vi "Cleanup.vi"(8 "error in (no error)":errorcluster, 11 "PlatformArrayPanel in":refnum<class "PlatformArrayPanel.lvclass">) -> (0 "error out":errorcluster)   [LabVIEW 2020, in "PicoG-App.lvlib" / "PlatformArrayPanel.lvclass"]
uses:
  PlatformArrayPanel.lvclass
  <vilib>/IlluminatedG/IG OOPanel/OOPanel/ArrayPanel/ArrayPanel.lvclass
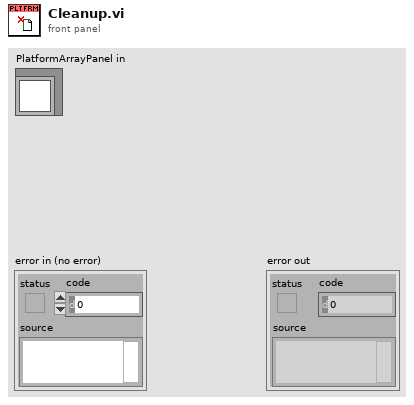
[diagram p1: front panel]
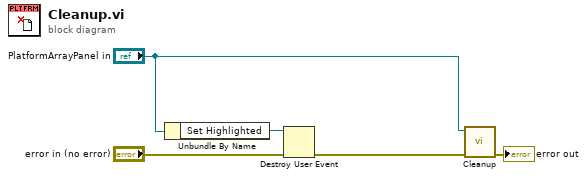
[diagram p0: block diagram]
diagram:
  n1 = Unbundle By Name("PlatformArrayPanel in") -> ("Set Highlighted"=w3:refnum<user-event>)
  n2 = Destroy User Event(user event=w3, error in="error in (no error)") -> (error out=w1:errorcluster)
  n3 = call-parent "Cleanup.vi"("error in (no error)"=w1, "ArrayPanel in"="PlatformArrayPanel in") -> ("error out"=→"error out":errorcluster)  [unwired: 9 in]
